vi "Multi_Stage_Resample.vi"(5 "X Resolution":i32, 7 "Y Resolution":i32, 8 "error in":errorcluster, 9 "Interpolation Type":u32(ring)=1 items=["Zero Order", "Bi-Linear", "Quadratic", "Cubic Spline"], 10 "Image Dest In":T1, 11 "Image Src":T1) -> (0 "error out":errorcluster, 3 "Img out":T1)   [LabVIEW 2020]
uses:
  <vilib>/vision/Image Controls.llb/IMAQ Image.ctl
  <vilib>/vision/NI_Vision_Development_Module.lvlib
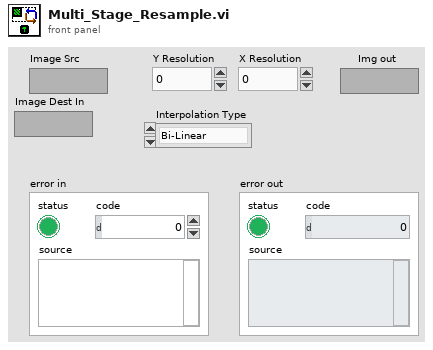
[diagram p1: front panel]
types:
  T1 = typedef "IMAQ Image.ctl" = refnum<image>
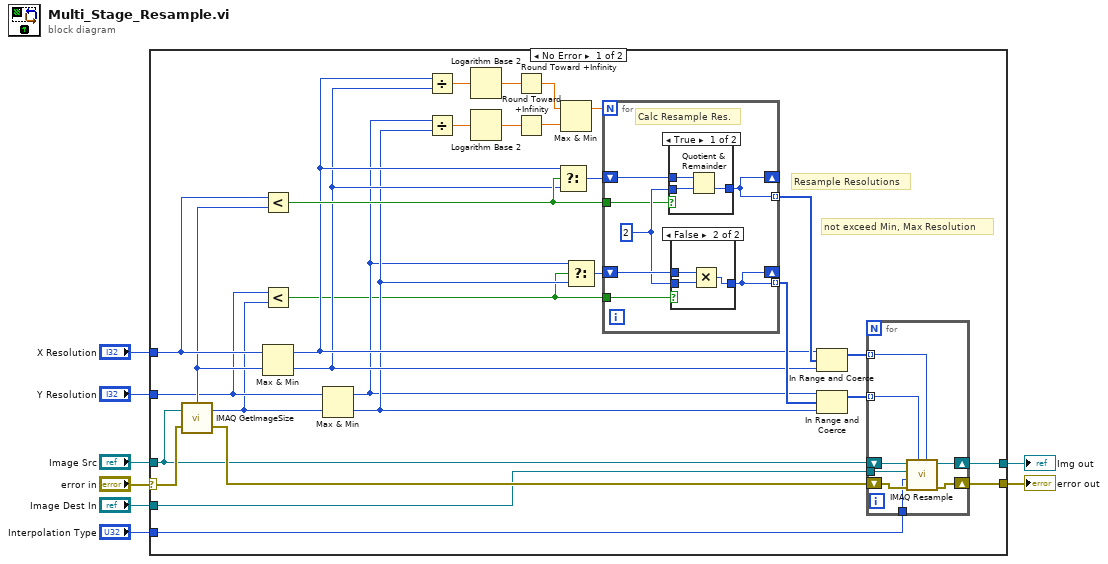
[diagram p0: block diagram]
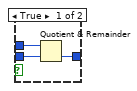
[diagram p2: hidden frame]
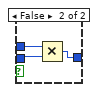
[diagram p3: hidden frame]
diagram:
  n1 = case shown="No Error" "error in" {
    selector: "error in" -> [w37 w66]
    tunnel: [w35 w66] -> w7
    tunnel: [w34 w67] -> w3
    tunnel: "Image Src" -> [w23 w67]
    tunnel: "Interpolation Type" -> [w22 _]
    tunnel: "Y Resolution" -> [w19 _]
    tunnel: "X Resolution" -> [w21 _]
    tunnel: "Image Dest In" -> [w9 _]
    frame No Error {
      # "Resample Resolutions"
      # "not exceed Min, Max Resolution"
      n2 = call "IMAQ GetImageSize"("Image"=w23, "error in (no error)"=w37) -> ("Y Resolution"=w18:i32, "X Resolution"=w20:i32, "error out"=w38:errorcluster)  [unwired: 2 in]
      n3 = Less?(x=w21, y=w20) -> (x < y?=w17:bool)
      n4 = Less?(x=w19, y=w18) -> (x < y?=w10:bool)
      n5 = Max & Min(x=w21, y=w20) -> (max(x,y)=w16:i32, min(x,y)=w15:i32)
      n6 = Max & Min(x=w19, y=w18) -> (max(x,y)=w12:i32, min(x,y)=w13:i32)
      n7 = Divide(x=w16, y=w15) -> (x/y=w32:dbl)
      n8 = Divide(x=w12, y=w13) -> (x/y=w30:dbl)
      n9 = Logarithm Base 2(1:w32) -> (0:w31:dbl)
      n10 = Logarithm Base 2(1:w30) -> (0:w33:dbl)
      n11 = Round Toward +Infinity(x=w31) -> (ceil(x): smallest int >= x=w29:dbl)
      n12 = Round Toward +Infinity(x=w33) -> (ceil(x): smallest int >= x=w36:dbl)
      n13 = Select(t=w16, s=w17, f=w15) -> (s? t:f=w14:i32)
      n14 = Max & Min(x=w29, y=w36) -> (max(x,y)=w28:dbl)  [unwired: 1 out]
      n15 = Select(t=w12, s=w10, f=w13) -> (s? t:f=w11:i32)
      n16 = for {
        N: w28 -> [_]
        tunnel: [w49] -> w27 mode=indexing
        tunnel: [w52] -> w26 mode=indexing
        shift-right: [w52] -> _
        shift-left: w14 -> [w53]
        shift-right: [w49] -> _
        shift-left: w11 -> [w51]
        tunnel: w17 -> [w48]
        tunnel: w10 -> [w47]
        w50 = 2 ("y")
        # "Calc Resample Res."
        n17 = case shown="True" w48 {
          tunnel: w53 -> [w62 w65]
          tunnel: [w61 w64] -> w52
          tunnel: w50 -> [w60 w63]
          frame True {
            n18 = Quotient & Remainder(x=w62, y=w60) -> (floor(x/y)=w61:i32)  [unwired: 1 out]
          }
          frame False {
            n19 = Multiply(x=w65, y=w63) -> (x*y=w64:i32)
          }
        }
        n20 = case shown="False" w47 {
          tunnel: w51 -> [w56 w59]
          tunnel: [w55 w58] -> w49
          tunnel: w50 -> [w54 w57]
          frame True {
            n21 = Quotient & Remainder(x=w56, y=w54) -> (floor(x/y)=w55:i32)  [unwired: 1 out]
          }
          frame False {
            n22 = Multiply(x=w59, y=w57) -> (x*y=w58:i32)
          }
        }
      }
      n23 = In Range and Coerce(upper limit=w16, x=w26, lower limit=w15) -> (coerced(x)=w25:i32[])  [unwired: 1 out]
      n24 = In Range and Coerce(upper limit=w12, x=w27, lower limit=w13) -> (coerced(x)=w24:i32[])  [unwired: 1 out]
      n25 = for {
        shift-right: [w45] -> w35
        shift-left: w38 -> [w46]
        shift-right: [w44] -> w34
        shift-left: w23 -> [w41]
        tunnel: w24 -> [w43] mode=indexing
        tunnel: w25 -> [w42] mode=indexing
        tunnel: w22 -> [w40]
        tunnel: w9 -> [w39]
        n26 = call "IMAQ Resample"("X Resolution"=w42, "Y Resolution"=w43, "error in (no error)"=w46, "Interpolation Type"=w40, "Image Dst"=w39, "Image Src"=w41) -> ("error out"=w45:errorcluster, "Image Dst Out"=w44:T1)  [unwired: 4 in]
      }
    }
    frame Error {
    }
  }
  "error out" <- w7
  "Img out" <- w3
